vi "Stop Driver Server.vi"(8 "error in (no error)":errorcluster) -> (0 "error out":errorcluster)   [LabVIEW 2010]
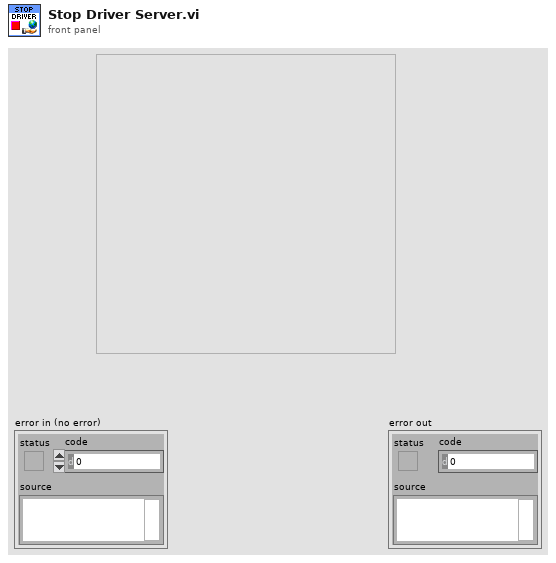
[diagram p1: front panel]
types:
  T1 = typedef "Path InitDynamicVIsPaths__FS.ctl" = cluster{"F4 Operation":path, "F4 Alarms":path, "F4 Inputs":path, "F4 Outputs":path, "F4 PID Sets":path, "F4 Cascade":path, "F4 Current Step":path, "Profile SubPanel":path, "Profile Editor":path, "MainVI":path, "Profile Control":path, "Synergy Control":path, "Driver Server":path}
  T2 = enum32{"Bad", "Idle", "Run top level", "Running"}
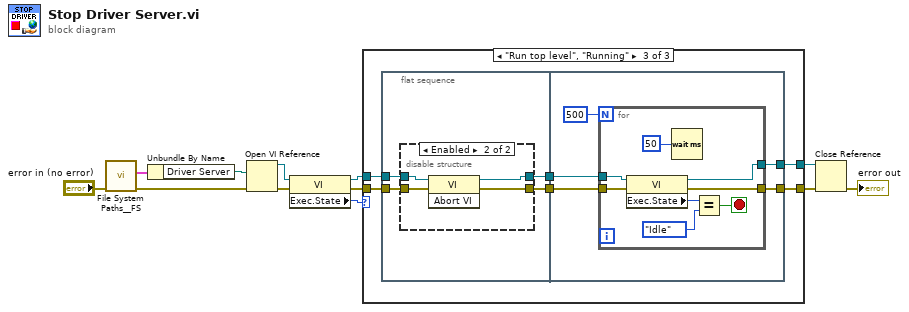
[diagram p0: block diagram]
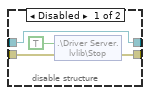
[diagram p4: hidden frame]
diagram:
  n1 = call "File System Paths__FS.vi"("error in (no error)"="error in (no error)") -> ("error out"=w6:errorcluster, "DynamicVIs"=w12:T1)  [unwired: 8 in, 1 out]
  n2 = Unbundle By Name(w12) -> ("Driver Server"=w11:path)
  n3 = Open VI Reference(vi path=w11, error in (no error)=w6) -> (vi reference=w10:refnum<vi>, error out=w5:errorcluster)  [unwired: 4 in]
  n4 = property class="VI"(reference=w10, error in=w5) -> (reference out=w8:refnum<vi>, error out=w4:errorcluster, "Exec.State"=w9:T2)
  n5 = case shown="\"Run top level\", \"Running\"" w9 {
    tunnel: [w14 w16 w21] -> w2
    tunnel: w4 -> [w14 w16 w20]
    tunnel: w8 -> [w13 w15 w18]
    tunnel: [w13 w15 w17] -> w3
    frame "Bad", Default {
    }
    frame "Idle" {
    }
    frame "Run top level", "Running" {
      n6 = flat-sequence {
        tunnel: [w25] -> w22
        tunnel: w20 -> [w26]
        tunnel: [w23] -> w19
        tunnel: w18 -> [w24]
        tunnel: w22 -> [w39]
        tunnel: [w38] -> w21
        tunnel: w19 -> [w36]
        tunnel: [w35] -> w17
        frame #0 {
          n7 = disable-structure shown="Enabled" {
            disable-tunnel: w26 -> [w29 w32]
            disable-tunnel: [w28 w31] -> w25
            disable-tunnel: w24 -> [w27 w34]
            disable-tunnel: [w27 w33] -> w23
            frame Disabled {
              n8 = shared-variable ".\\Driver Server.lvlib\\Stop"(TRUE ("Stop"), error in=w29) -> (error out=w28:errorcluster)
            }
            frame Enabled {
              n9 = invoke class="VI" method="Abort VI"(reference=w34, error in=w32) -> (reference out=w33:refnum<vi>, error out=w31:errorcluster)  [unwired: 1 in, 1 out]
            }
          }
        }
        frame #1 {
          n10 = for {
            N: 500 -> [_]
            tunnel: w39 -> [w42]
            tunnel: [w41] -> w38
            tunnel: w36 -> [w46]
            tunnel: [w40] -> w35
            stop <- w43 stop-if-true
            n11 = property class="VI"(reference=w46, error in=w42) -> (reference out=w40:refnum<vi>, error out=w41:errorcluster, "Exec.State"=w45:T2)
            n12 = Wait (ms)(milliseconds to wait=u32 50) -> ()  [unwired: 1 out]
            n13 = Equal?(x=w45, y=T2."Idle") -> (x = y?=w43:bool)
          }
        }
      }
    }
  }
  n14 = Close Reference(reference=w3, error in (no error)=w2) -> (error out=→"error out":errorcluster)
